vi "SMTP Email RFC-1123 Date.vi"(0 "time (now)":dbl format="%0.2f", 1 "numeric zone offset (true)":bool=TRUE) -> (2 "GMT Date/Time":string)   [LabVIEW 2012, in "NewNI_SMTPEmail.lvlib"]
doc: "Formats time according to RFC-1123.\n\ntime - time to be formated (defaults to current time)\n\nnumeric zone offset -\n if TRUE, formats to local time with GMT offset\n if FALSE, formats to GMT time"
uses:
  NewNI_SMTPEmail.lvlib
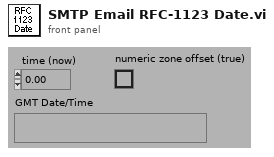
[diagram p1: front panel]
types:
  T1 = cluster{"second":i32, "minute":i32, "hour":i32, "day of month":i32, "month":i32, "year":i32, "day of week":i32, "day of year":i32, "is DST":i32}
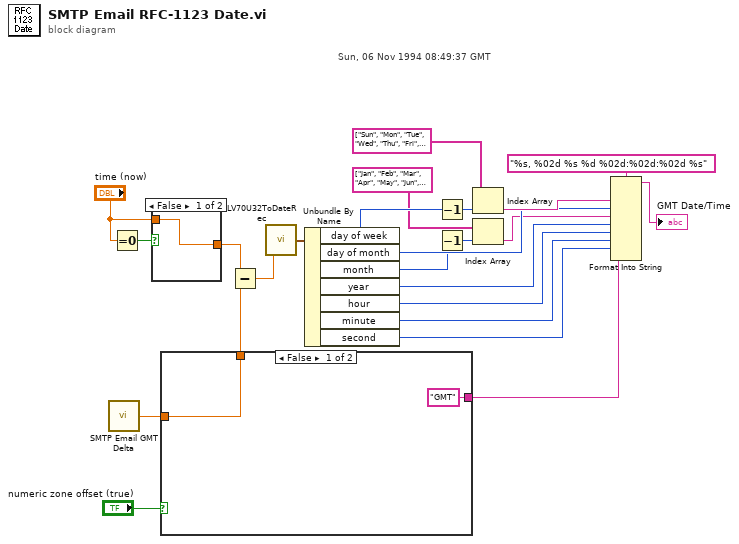
[diagram p0: block diagram]
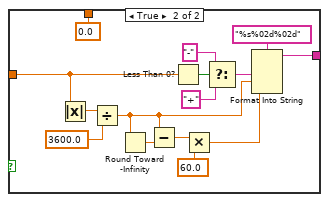
[diagram p2: hidden frame]
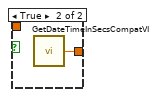
[diagram p3: hidden frame]
diagram:
  # "Sun, 06 Nov 1994 08:49:37 GMT"
  n1 = call "SMTP Email GMT Delta.vi"() -> ("GMT Delta in seconds"=w2:dbl)
  n2 = Equal To 0?(x="time (now)") -> (x = 0?=w6:bool)
  n3 = case shown="False" w6 {
    tunnel: [w25 w26] -> w8
    tunnel: "time (now)" -> [w25 _]
    frame False {
    }
    frame True {
      n4 = call <vilib>:"GetDateTimeInSecsCompatVI.vi"() -> ("double precision float"=w26:dbl)  [unwired: 1 out]
    }
  }
  n5 = case shown="False" "numeric zone offset (true)" {
    tunnel: ["GMT" w40] -> w4
    tunnel: w2 -> [w27 w38]
    tunnel: [w27 0.0 ("GMT Delta in seconds")] -> w1
    frame False {
    }
    frame True {
      n6 = Absolute Value(x=w38) -> (abs(x)=w37:dbl)
      n7 = Divide(x=w37, y=3600.0) -> (x/y=w41:dbl)
      n8 = Round Toward -Infinity(1:w41) -> (0:w34:dbl)
      n9 = Subtract(x=w41, y=w34) -> (x-y=w35:dbl)
      n10 = Less Than 0?(x=w38) -> (x < 0?=w31:bool)
      n11 = Multiply(x=w35, y=60.0) -> (x*y=w42:dbl)
      n12 = Select(t="-", s=w31, f="+") -> (s? t:f=w43:string)
      n13 = Format Into String(format string="%s%02d%02d", w43, w41, w42) -> (resulting string=w40:string)  [unwired: 2 in, 1 out]
    }
  }
  n14 = Subtract(x=w8, y=w1) -> (x-y=w7:dbl)
  n15 = call <vilib>:"LV70U32ToDateRec.vi"("Time"=w7) -> ("date time rec"=w20:T1)
  n16 = Unbundle By Name(w20) -> ("day of week"=w19:i32, "day of month"=w18:i32, "month"=w10:i32, "year"=w17:i32, "hour"=w16:i32, "minute"=w15:i32, "second"=w14:i32)
  n17 = Decrement(x=w19) -> (x-1=w22:i32)
  n18 = Decrement(x=w10) -> (x-1=w11:i32)
  n19 = Index Array(array=string[] ["Sun", "Mon", "Tue", "Wed", "Thu", "Fri", "Sat"], index=w22) -> (element=w21:string)
  n20 = Index Array(array=string[] ["Jan", "Feb", "Mar", "Apr", "May", "Jun", "Jul", "Aug", "Sep", "Oct", "Nov", "Dec"], index=w11) -> (element=w13:string)
  n21 = Format Into String(format string="%s, %02d %s %d %02d:%02d:%02d %s", w21, w18, w13, w17, w16, w15, w14, w4) -> (resulting string=→"GMT Date/Time":string)  [unwired: 2 in, 1 out]
